vi "ModifyGraph rgb.vi"(8 "error in (no error)":errorcluster, 10 "Colorscale":u32[](array[colorbox])=[16711680, 16744448, 16776960, 65280, 255, 8388863, 16711935], 11 "ITX Commands in":refnum<class "ITX Commands.lvclass">) -> (0 "error out":errorcluster, 3 "ITX Commands out":refnum<class "ITX Commands.lvclass">)   [LabVIEW 2016, in "ITX Commands.lvclass"]
uses:
  ITX Commands.lvclass
  ITX Commands.lvclass/ITX Commands.ctl
  <userlib>/LevyLab/Graph Utilities/graph_utilities.lvclass
panel:
  out "delimited string":string
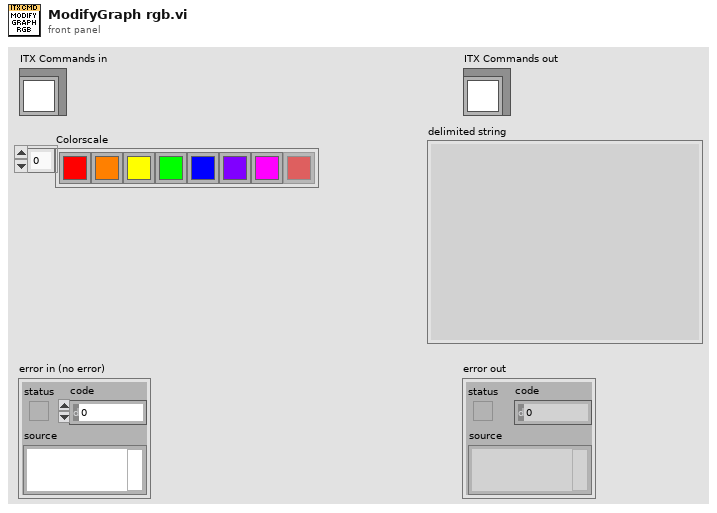
[diagram p1: front panel]
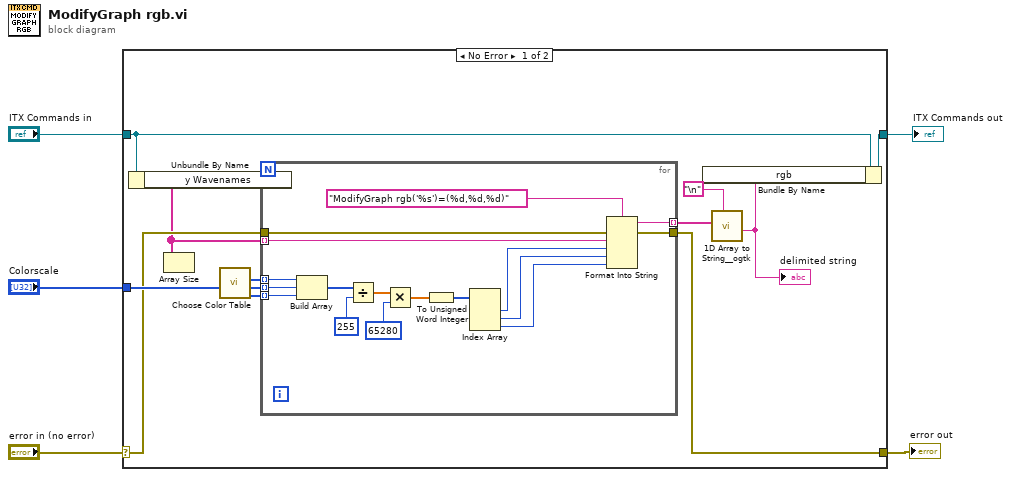
[diagram p0: block diagram]
diagram:
  n1 = case shown="No Error" "error in (no error)" {
    selector: "error in (no error)" -> [w9 w36]
    tunnel: [w8 w36] -> w4
    tunnel: [w14 w35] -> w2
    tunnel: "ITX Commands in" -> [w7 w35]
    tunnel: "Colorscale" -> [w10 _]
    frame No Error {
      n2 = Unbundle By Name(w7) -> ("y Wavenames"=w6:string[])
      n3 = Array Size(array=w6) -> ()  [unwired: 1 out]
      n4 = call <userlib>:"Choose Color Table.vi"("Custom Table"=w10) -> ("B []"=w15:u8[], "G []"=w16:u8[], "R []"=w17:u8[])  [unwired: 7 in, 1 out]
      n5 = for {
        tunnel: w17 -> [w29] mode=indexing
        tunnel: w16 -> [w28] mode=indexing
        tunnel: w15 -> [w27] mode=indexing
        tunnel: [w25] -> w12 mode=indexing
        tunnel: w6 -> [w24] mode=indexing
        tunnel: w9 -> [w19]
        tunnel: [w18] -> w8
        n6 = Build Array(w29, w28, w27) -> (w30:u8[])
        n7 = Divide(x=w30, y=255) -> (x/y=w31:dbl[])
        n8 = Multiply(x=w31, y=65280) -> (x*y=w32:dbl[])
        n9 = To Unsigned Word Integer(number=w32) -> (unsigned 16bit integer=w23:u16[])
        n10 = Index Array(array=w23) -> (element #1=w22:u16, element #2=w21:u16, element #3=w20:u16)  [unwired: 3 in]
        n11 = Format Into String(format string="ModifyGraph rgb('%s')=(%d,%d,%d)", error in=w19, w24, w22, w21, w20) -> (resulting string=w25:string, error out=w18:errorcluster)  [unwired: 1 in]
      }
      n12 = call <userlib>:"1D Array to String__ogtk.vi"("delimiter (Tab)"="\n", "Array of Strings"=w12) -> ("delimited string"=w11:string)  [unwired: 9 in]
      "delimited string" <- w11
      n13 = Bundle By Name(cluster=w7, "rgb"=w11) -> (w14:refnum<class "ITX Commands.lvclass">)
    }
    frame Error {
    }
  }
  "error out" <- w4
  "ITX Commands out" <- w2
